vi "messaging_processor_handler.vi"(0 "actions":T3[](array[typedef]), 1 "interaction_descriptors (in)":T2[](array[typedef]), 2 "params":T1, 5 "error in (no error)":errorcluster) -> (19 "error out":errorcluster)   [LabVIEW 2016]
uses:
  controls/messaging_processor_handler_actions.ctl
  pre-build/support/controls/raw_object_interaction_descriptor.ctl
  controls/messaging_processor_params.ctl
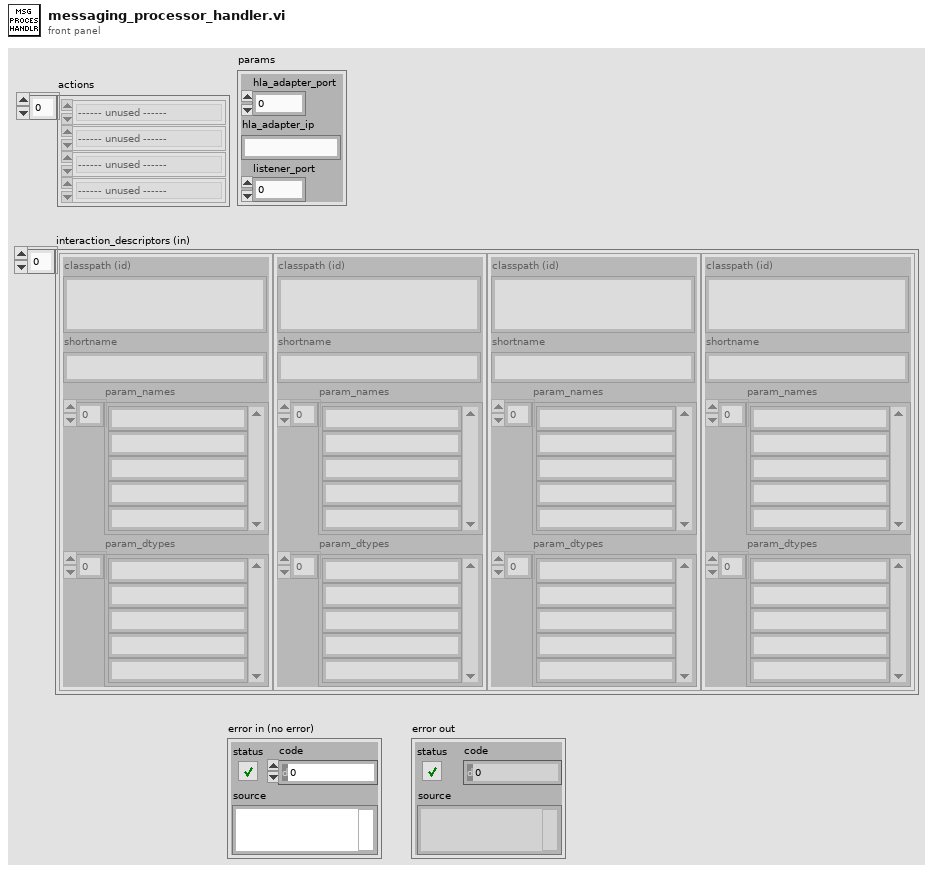
[diagram p1: front panel]
types:
  T1 = typedef "messaging_processor_params.ctl" = cluster{"hla_adapter_port":u16, "hla_adapter_ip":string, "listener_port":u16}
  T2 = typedef "raw_object_interaction_descriptor.ctl" = cluster{"classpath (id)":string, "shortname":string, "param_names":string[], "param_dtypes":string[]}
  T3 = typedef "messaging_processor_handler_actions.ctl" = enum16{"------ unused ------", "close", "init", "launch", "run"}
  T4 = enum32{"invalid app kind", "Development System", "Run Time System", "Student Edition", "Embedded LabVIEW", "Evaluation", "Custom"}
  T5 = enum32{"Invalid", "Standard", "Closed", "Hidden", "Minimized", "Maximized"}
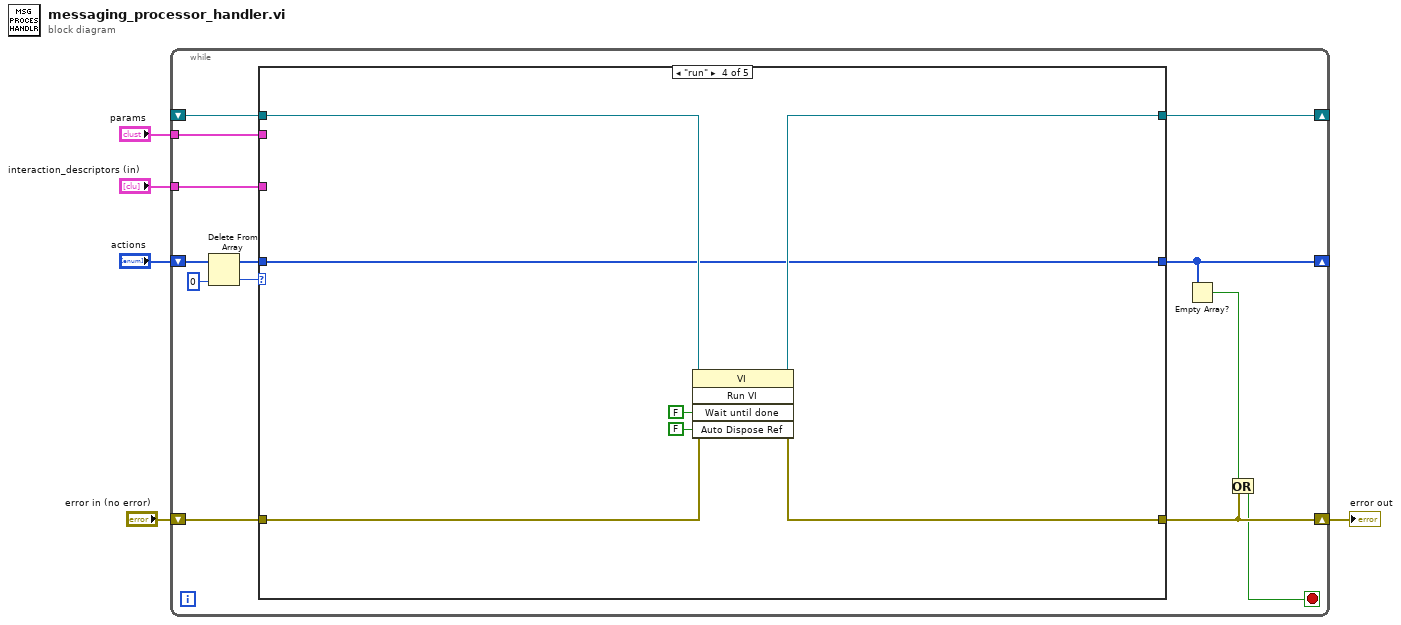
[diagram p0: block diagram]
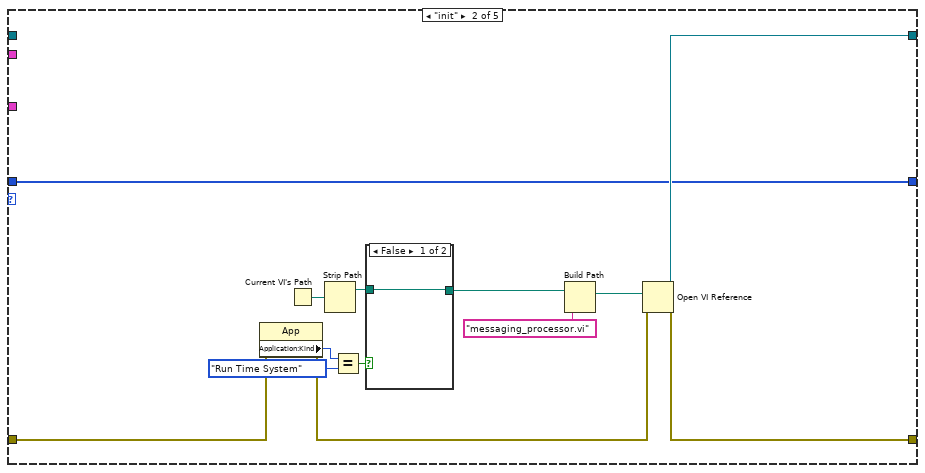
[diagram p3: hidden frame]
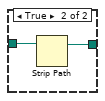
[diagram p4: hidden frame]
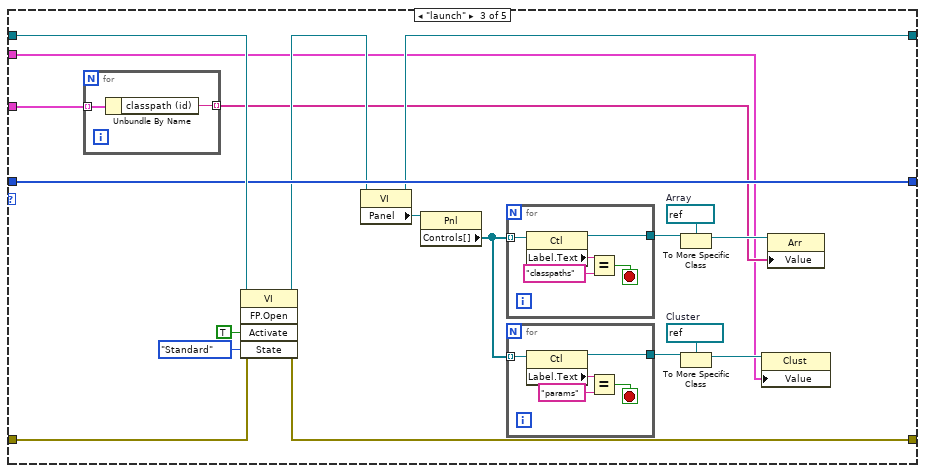
[diagram p5: hidden frame]
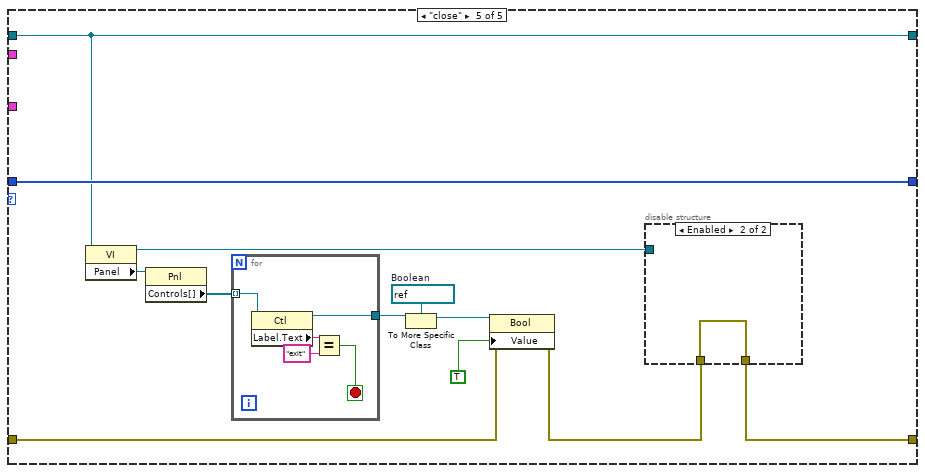
[diagram p6: hidden frame]
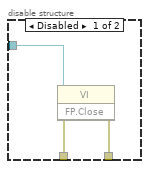
[diagram p7: hidden frame]
diagram:
  n1 = while {
    shift-right: [w11] -> _
    shift-left: "actions" -> [w18]
    shift-right: [w9] -> w3
    shift-left: "error in (no error)" -> [w15]
    shift-right: [w14] -> _
    shift-left: _ -> [w12]
    tunnel: "interaction_descriptors (in)" -> [w7]
    tunnel: "params" -> [w6]
    stop <- w8 stop-if-true
    n2 = Delete From Array(array=w18, index=0) -> (deleted portion=w16:T3, array with subset deleted=w13:T3[])  [unwired: 1 in]
    n3 = case shown="\"run\"" w16 {
      tunnel: w15 -> [w19 w29 w53 w74 w79]
      tunnel: [w19 w24 w51 w71 w76] -> w9
      tunnel: [w21 w23 w45 w73 w80] -> w14
      tunnel: w13 -> [w20 w22 w52 w72 w87]
      tunnel: [w20 w22 w52 w72 w87] -> w11
      tunnel: w12 -> [w21 _ w56 w75 w80]
      tunnel: w7 -> [_ _ w50 _ _]
      tunnel: w6 -> [_ _ w38 _ _]
      frame "------ unused ------", Default {
      }
      frame "init" {
        n4 = property on="Property Node" class="App"(error in=w29) -> (error out=w25:errorcluster, "Application:Kind"=w33:T4)  [unwired: 1 in, 1 out]
        n5 = Current VI's Path() -> (path=w34:path)
        n6 = Strip Path(path=w34) -> (stripped path=w30:path)  [unwired: 1 out]
        n7 = Equal?(x=w33, y=T4."Run Time System") -> (x = y?=w31:bool)
        n8 = case shown="False" w31 {
          tunnel: w30 -> [w35 w37]
          tunnel: [w35 w36] -> w28
          frame False {
          }
          frame True {
            n9 = Strip Path(path=w37) -> (stripped path=w36:path)  [unwired: 1 out]
          }
        }
        n10 = Build Path(base path=w28, name or relative path="messaging_processor.vi") -> (appended path=w26:path)
        n11 = Open VI Reference(vi path=w26, error in (no error)=w25) -> (vi reference=w23:refnum<vi>, error out=w24:errorcluster)  [unwired: 4 in]
      }
      frame "launch" {
        w40 = refnum<vi> refnum  # Cluster
        w47 = refnum<vi> refnum  # Array
        n12 = for {
          tunnel: w50 -> [w68] mode=indexing
          tunnel: [w67] -> w43 mode=indexing
          n13 = Unbundle By Name(w68) -> ("classpath (id)"=w67:string)
        }
        n14 = invoke class="VI" method="FP.Open"(reference=w56, error in=w53, "Activate"=TRUE ("Activate?"), "State"=T5."Standard") -> (reference out=w46:refnum<vi>, error out=w51:errorcluster)  [unwired: 1 in, 3 out]
        n15 = property class="VI"(reference=w46) -> (reference out=w45:refnum<vi>, "Panel"=w49:refnum<vi>)  [unwired: 1 in, 1 out]
        n16 = property class="Pnl"(reference=w49) -> ("Controls[]"=w42:refnum<vi>[])  [unwired: 1 in, 2 out]
        n17 = for {
          tunnel: w42 -> [w66] mode=indexing
          tunnel: [w62] -> w48
          stop <- w63 stop-if-true
          n18 = property class="Ctl"(reference=w66) -> (reference out=w62:refnum<vi>, "Label.Text"=w65:string)  [unwired: 1 in, 1 out]
          n19 = Equal?(x=w65, y="classpaths") -> (x = y?=w63:bool)
        }
        n20 = for {
          tunnel: w42 -> [w61] mode=indexing
          tunnel: [w57] -> w39
          stop <- w58 stop-if-true
          n21 = property class="Ctl"(reference=w61) -> (reference out=w57:refnum<vi>, "Label.Text"=w60:string)  [unwired: 1 in, 1 out]
          n22 = Equal?(x=w60, y="params") -> (x = y?=w58:bool)
        }
        n23 = To More Specific Class(target class=w47, reference=w48) -> (specific class reference=w44:refnum<vi>)  [unwired: 1 in, 1 out]
        n24 = To More Specific Class(target class=w40, reference=w39) -> (specific class reference=w41:refnum<vi>)  [unwired: 1 in, 1 out]
        n25 = property class="Clust"(reference=w41, "Value"=w38) -> ()  [unwired: 1 in, 2 out]
        n26 = property class="Arr"(reference=w44, "Value"=w43) -> ()  [unwired: 1 in, 2 out]
      }
      frame "run" {
        n27 = invoke class="VI" method="Run VI"(reference=w75, error in=w74, "Wait until done"=FALSE ("Wait Until Done"), "Auto Dispose Ref"=FALSE ("Auto Dispose Reference")) -> (reference out=w73:refnum<vi>, error out=w71:errorcluster)  [unwired: 1 in, 3 out]
      }
      frame "close" {
        w83 = refnum<vi> refnum  # Boolean
        n28 = property class="VI"(reference=w80) -> (reference out=w78:refnum<vi>, "Panel"=w86:refnum<vi>)  [unwired: 1 in, 1 out]
        n29 = property class="Pnl"(reference=w86) -> ("Controls[]"=w85:refnum<vi>[])  [unwired: 1 in, 2 out]
        n30 = for {
          tunnel: w85 -> [w96] mode=indexing
          tunnel: [w92] -> w84
          stop <- w93 stop-if-true
          n31 = property class="Ctl"(reference=w96) -> (reference out=w92:refnum<vi>, "Label.Text"=w95:string)  [unwired: 1 in, 1 out]
          n32 = Equal?(x=w95, y="exit") -> (x = y?=w93:bool)
        }
        n33 = To More Specific Class(target class=w83, reference=w84) -> (specific class reference=w82:refnum<vi>)  [unwired: 1 in, 1 out]
        n34 = property class="Bool"(reference=w82, error in=w79, "Value"=TRUE) -> (error out=w77:errorcluster)  [unwired: 1 out]
        n35 = disable-structure shown="Enabled" {
          disable-tunnel: w78 -> [w90 _]
          disable-tunnel: w77 -> [w89 w91]
          disable-tunnel: [w88 w91] -> w76
          frame Disabled {
            n36 = invoke class="VI" method="FP.Close"(reference=w90, error in=w89) -> (error out=w88:errorcluster)  [unwired: 1 in, 2 out]
          }
          frame Enabled {
          }
        }
      }
    }
    n37 = Empty Array?(array=w11) -> (empty?=w10:bool)
    n38 = Or(x=w10, y=w9) -> (x .or. y?=w8:bool)
  }
  "error out" <- w3
